vi "Meas Proc QWTB Load Result Spectra.vi"(7 "phase ref":refnum<vi>, 8 "error in":errorcluster, 11 "meas root":path) -> (0 "error out":errorcluster, 3 "graphs":T1[](array[typedef]))   [LabVIEW 2020]
uses:
  Meas Proc QWTB Spectrum Data.ctl
  octave/infolib/GetString.vi
  octave/infolib/Get 1D String.vi
  octave/infolib/GetI64.vi
  octave/infolib/Get 2D String.vi
  octave/infolib/infolib.lvlib
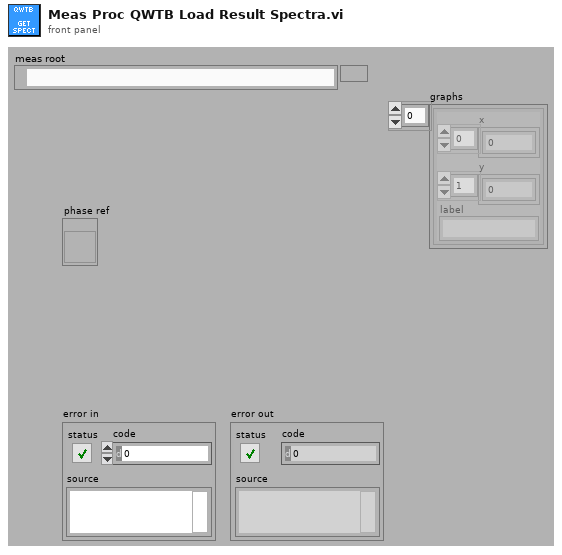
[diagram p1: front panel]
types:
  T1 = typedef "Meas Proc QWTB Spectrum Data.ctl" = cluster{"x":sgl[], "y":sgl[], "label":string}
  T2 = typedef "MAT Type Representation.ctl" = enum16{"DBL", "SGL", "I32", "I16", "U16", "U8", "CDB", "CSG", "STR"}
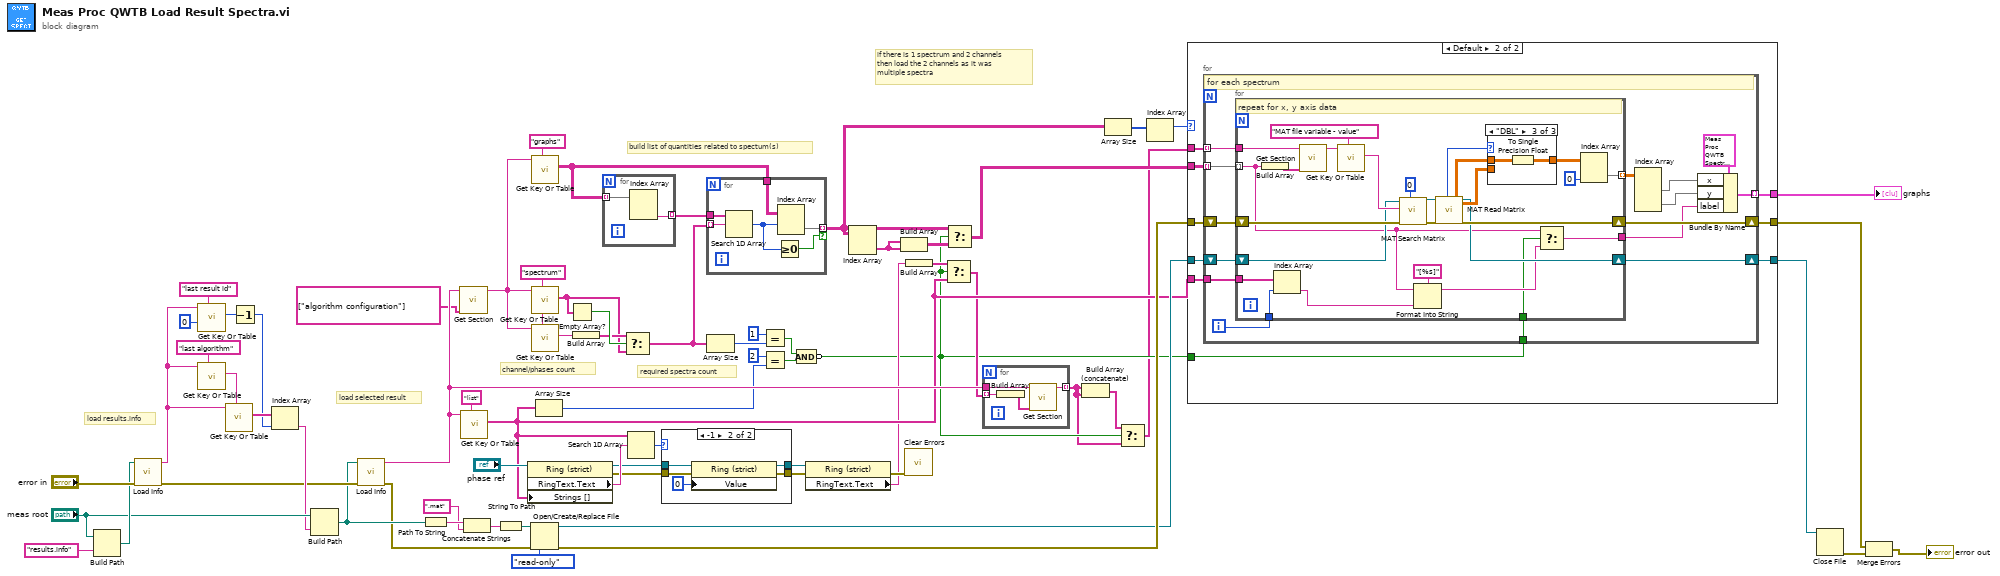
[diagram p0: block diagram]
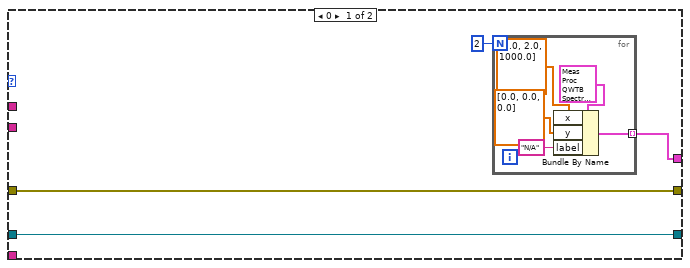
[diagram p2: hidden frame]
diagram:
  w28 = "spectrum" ("key description")
  # "if there is 1 spectrum and 2 channels\nthen load the 2 channels as it was\nmultiple spectra"
  # "channel/phases count"
  # "required spectra count"
  # "load selected result"
  # "load results.info"
  # "build list of quantities related to spectum(s)"
  n1 = Build Path(base path="meas root", name or relative path="results.info") -> (appended path=w59:path)
  n2 = call "Load Info.vi"("error in"="error in", "filename"=w59) -> ("error out"=w56:errorcluster, "info data"=w64:string)  [unwired: 8 in]
  n3 = call-poly "Get Key Or Table.vi"("key description"="last result id", "numeric"=i64 0, "info data"=w64) -> ("value"=w62:i64)  [unwired: 5 in, 3 out]
  n4 = call-poly "Get Key Or Table.vi"("key description"="last algorithm", "info data"=w64) -> ("value"=w65:string)  [unwired: 6 in, 3 out]
  n5 = call-poly "Get Key Or Table.vi"("key description"=w65, "info data"=w64) -> ("value"=w63:string[])  [unwired: 6 in, 3 out]
  n6 = Decrement(x=w62) -> (x-1=w61:i64)
  n7 = Index Array(array=w63, index=w61) -> (element=w57:string)
  n8 = Build Path(base path="meas root", name or relative path=w57) -> (appended path=w42:path)
  n9 = call "Load Info.vi"("error in"=w56, "filename"=w42) -> ("error out"=w37:errorcluster, "info data"=w45:string)  [unwired: 8 in]
  n10 = Path To String(path=w42) -> (string=w41:string)
  n11 = call "Get Section.vi"("sections"=string[] ["algorithm configuration"], "info data"=w45) -> ("section part"=w27:string)  [unwired: 7 in, 2 out]
  n12 = call-poly "Get Key Or Table.vi"("key description"="list", "info data"=w45) -> ("value"=w12:string[])  [unwired: 6 in, 3 out]
  n13 = Concatenate Strings(w41, ".mat" ("name or relative path")) -> (w39:string)
  n14 = String To Path(string=w39) -> (path=w38:path)
  n15 = property class="Ring (strict)"(reference="phase ref", "Strings []"=w12) -> (reference out=w50:refnum<vi>, error out=w49:errorcluster, "RingText.Text"=w52:string)  [unwired: 1 in]
  n16 = Open/Create/Replace File(file path (use dialog)=w38, error in=w37, access (0:read/write)=enum16{"read/write", "read-only", "write-only"}."read-only") -> (refnum out=w33:refnum<file>, error out=w35:errorcluster)  [unwired: 3 in, 1 out]
  n17 = call-poly "Get Key Or Table.vi"("key description"="graphs", "info data"=w27) -> ("value"=w43:string[][])  [unwired: 6 in, 3 out]
  n18 = call-poly "Get Key Or Table.vi"("key description"=w28, "info data"=w27) -> ("value"=w23:string[])  [unwired: 6 in, 3 out]
  n19 = call-poly "Get Key Or Table.vi"("key description"=w28, "info data"=w27) -> ("value"=w25:string)  [unwired: 6 in, 3 out]
  n20 = Array Size(array=w12) -> (size(s)=w21:i32)
  n21 = Empty Array?(array=w23) -> (empty?=w26:bool)
  n22 = Build Array(w25) -> (w24:string[])
  n23 = for {
    tunnel: w43 -> [w71] mode=indexing
    tunnel: [w70] -> w44 mode=indexing
    n24 = Index Array(array=w71) -> (element #2=w70:string)  [unwired: 2 in, 1 out]
  }
  n25 = Select(t=w24, s=w26, f=w23) -> (s? t:f=w22:string[])
  n26 = Search 1D Array(1D array=w12, element=w52) -> (index of element=w51:i32)  [unwired: 1 in]
  n27 = case shown="-1" w51 {
    tunnel: w50 -> [w73 w78]
    tunnel: w49 -> [w72 w76]
    tunnel: [w72 w75] -> w48
    tunnel: [w73 w74] -> w47
    frame Default {
    }
    frame -1 {
      n28 = property class="Ring (strict)"(reference=w78, error in=w76, "Value"=u16 0) -> (reference out=w74:refnum<vi>, error out=w75:errorcluster)
    }
  }
  n29 = for {
    tunnel: w22 -> [w83] mode=indexing
    tunnel: w44 -> [w84]
    tunnel: w43 -> [w82]
    tunnel: [w81] -> w2 mode=indexing if=w80
    n30 = Search 1D Array(1D array=w84, element=w83) -> (index of element=w79:i32)  [unwired: 1 in]
    n31 = Greater Or Equal To 0?(x=w79) -> (x >= 0?=w80:bool)
    n32 = Index Array(array=w82, index (row)=w79) -> (element=w81:string[])  [unwired: 1 in]
  }
  n33 = Array Size(array=w22) -> (size(s)=w19:i32)
  n34 = Equal?(x=1, y=w19) -> (x = y?=w16:bool)
  n35 = Equal?(x=2, y=w21) -> (x = y?=w17:bool)
  n36 = Compound Arithmetic op=AND(w16, w17) -> (invert w8:bool)
  n37 = property class="Ring (strict)"(reference=w47, error in=w48) -> (error out=w46:errorcluster, "RingText.Text"=w11:string)  [unwired: 1 out]
  n38 = Index Array(array=w2) -> (element=w13:string[])  [unwired: 2 in]
  n39 = Build Array(w13, w13) -> (w15:string[][])
  n40 = call <vilib>:"Clear Errors.vi"("error in (no error)"=w46) -> ()  [unwired: 5 in, 2 out]
  n41 = Build Array(w11) -> (w10:string[])
  n42 = Select(t=w10, s=w8, f=w12) -> (s? t:f=w9:string[])
  n43 = Select(t=w2, s=w8, f=w15) -> (s? t:f=w14:string[][])
  n44 = for {
    tunnel: w9 -> [w88] mode=indexing
    tunnel: w45 -> [w87]
    tunnel: [w86] -> w6 mode=indexing
    n45 = Build Array(w88) -> (w85:string[])
    n46 = call "Get Section.vi"("sections"=w85, "info data"=w87) -> ("section part"=w86:string)  [unwired: 7 in, 2 out]
  }
  n47 = Build Array (concatenate)(w6, w6) -> (w7:string[])
  n48 = Array Size(array=w2) -> (size(s)=w3:i32[])
  n49 = Select(t=w7, s=w8, f=w6) -> (s? t:f=w4:string[])
  n50 = Index Array(array=w3) -> (element=w1:i32)  [unwired: 1 in]
  n51 = case shown="Default" w1 {
    tunnel: w35 -> [w92 w106]
    tunnel: [w90 w105] -> w34
    tunnel: w33 -> [w91 w104]
    tunnel: [w91 w103] -> w32
    tunnel: [w92 w102] -> w29
    tunnel: w14 -> [_ w101]
    tunnel: w12 -> [_ w100]
    tunnel: w8 -> [_ w99]
    tunnel: w4 -> [_ w98]
    frame 0 {
      n52 = for {
        N: 2 -> [_]
        tunnel: [w96] -> w90 mode=indexing
        n53 = Bundle By Name(cluster=T1 {"x"=array[24001 elements], "y"=array[24001 elements], "label"=""} ("Meas Proc QWTB Spectrum Data"), "x"=sgl[] [1.0, 2.0, 1000.0], "y"=sgl[] [0.0, 0.0, 0.0] ("x"), "label"="N/A") -> (w96:T1)
      }
    }
    frame Default {
      n54 = for {
        tunnel: w101 -> [w121] mode=indexing
        tunnel: w98 -> [w120] mode=indexing
        shift-right: [w119] -> w102
        shift-left: w106 -> [w118]
        tunnel: [w114] -> w105 mode=indexing
        shift-right: [w110] -> w103
        shift-left: w104 -> [w111]
        tunnel: w100 -> [w108]
        tunnel: w99 -> [w107]
        i -> [w109]
        # "for each spectrum"
        n55 = for {
          tunnel: w121 -> [w124] mode=indexing
          tunnel: w120 -> [w147]
          shift-right: [w140] -> w119
          shift-left: w118 -> [w139]
          tunnel: [w133] -> w117 mode=indexing
          tunnel: [w130] -> w112
          shift-right: [w131] -> w110
          shift-left: w111 -> [w132]
          tunnel: w109 -> [w127]
          tunnel: w108 -> [w126]
          tunnel: w107 -> [w123]
          # "repeat for x, y axis data"
          n56 = Build Array(w124) -> (w122:string[])
          n57 = Index Array(array=w126, index=w127) -> (element=w125:string)
          n58 = call "Get Section.vi"("sections"=w122, "info data"=w147) -> ("section part"=w146:string)  [unwired: 7 in, 2 out]
          n59 = call-poly "Get Key Or Table.vi"("key description"="MAT file variable - value", "info data"=w146) -> ("value"=w144:string)  [unwired: 6 in, 3 out]
          n60 = call "MAT Search Matrix.vi"("offset in (-1: current position)"=i64 0, "Error In"=w139, "matrix name"=w144, "Ref Num"=w132) -> ("error out"=w142:errorcluster, "Dup Ref Num"=w141:refnum<file>)  [unwired: 6 in]
          n61 = Format Into String(format string="[%s]", initial string=w124, w125) -> (resulting string=w128:string)  [unwired: 1 in, 1 out]
          n62 = call "MAT Read Matrix.vi"("Ref Num"=w141, "Error In"=w142) -> ("Representation"=w138:T2, "DBL"=w136:dbl[][], "Dup Ref Num"=w131:refnum<file>, "SGL"=w137:sgl[][], "error out"=w140:errorcluster)  [unwired: 5 in, 8 out]
          n63 = case shown="\"DBL\"" w138 {
            tunnel: w137 -> [w148 _ _]
            tunnel: w136 -> [_ _ w150]
            tunnel: [w148 _ w149] -> w135
            frame "SGL" {
            }
            frame Default {
            }
            frame "DBL" {
              n64 = To Single Precision Float(number=w150) -> (single precision float=w149:sgl[][])
            }
          }
          n65 = Select(t=w124, s=w123, f=w128) -> (s? t:f=w130:string)
          n66 = Index Array(array=w135, index (col)=0 ("disabled index (col)")) -> (element=w133:sgl[])  [unwired: 1 in]
        }
        n67 = Index Array(array=w117) -> (element #1=w116:sgl[], element #2=w115:sgl[])  [unwired: 4 in]
        n68 = Bundle By Name(cluster=T1 {"x"=array[24001 elements], "y"=array[24001 elements], "label"=""} ("Meas Proc QWTB Spectrum Data"), "x"=w116, "y"=w115, "label"=w112) -> (w114:T1)
      }
    }
  }
  "graphs" <- w34
  n69 = Close File(refnum=w32) -> (error out=w31:errorcluster)  [unwired: 1 in, 1 out]
  n70 = Merge Errors(w29, w31) -> (→"error out":errorcluster)
